vi "fake prompt concatanate strings.vi"(9 "input 3":string, 10 "input 2":string, 11 "input 1":string) -> (3 "resulting string":string)   [LabVIEW 2020, in "MCP Server tests.lvlib"]
uses:
  MCP Server tests.lvlib
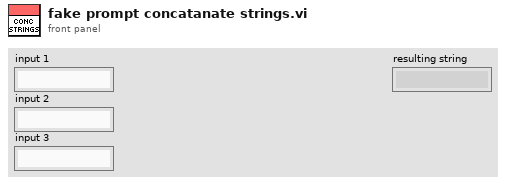
[diagram p1: front panel]
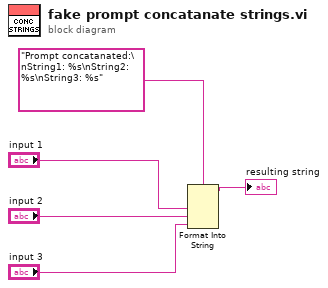
[diagram p0: block diagram]
diagram:
  n1 = Format Into String(format string="Prompt concatanated:\nString1: %s\nString2: %s\nString3: %s", "input 1", "input 2", "input 3") -> (resulting string=→"resulting string":string)  [unwired: 2 in, 1 out]
